vi "set active element.vi"(8 "error in (no error)":errorcluster, 11 "elem":string) -> (0 "error out":errorcluster)   [LabVIEW 2019, in "libSimulationControl.lvlib"]
doc: "void set_active_element(const char* elem);"
uses:
  libSimulationControl.lvlib
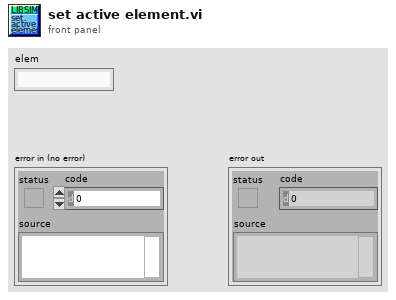
[diagram p1: front panel]
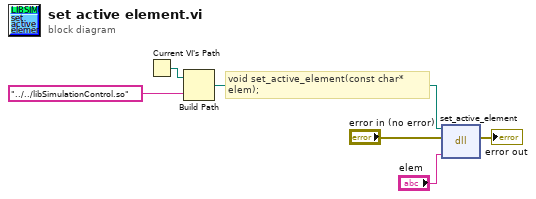
[diagram p0: block diagram]
diagram:
  # "void set_active_element(const char* elem);"
  n1 = Current VI's Path() -> (path=w3:path)
  n2 = Build Path(base path=w3, name or relative path="../../libSimulationControl.so") -> (appended path=w1:path)
  n3 = dll-call lib="home/paul/Schreibtisch/Biogas_plant_setup/LabView/lib/libSimulationControl/libSimulationControl.*" fn="set_active_element"(path in=w1, error in="error in (no error)", "elem"="elem") -> (error out=→"error out":errorcluster)  [unwired: 3 in, 1 out]
